vi "ncmainui.vi"() -> ()   [LabVIEW 2011]
uses:
  API/API DYM.lvlib
panel:
  in  "气缸":enum16{"向上", "向下"}(ring)
  in  "回参考点":bool
  out "CodeLine":i32
  out "CurrnetY":dbl
  out "CurrentX":dbl
  in  "撤消指令":bool
  in  "清空列表":bool
  in  "保存列表":bool
  in  "打开列表":bool
  in  "紧急停止":bool
  in  "开始执行":bool
  in  "选择坐标系统":enum32{"相对坐标", "绝度坐标"}(radio)
  in  "CodeList":i32(listbox)
  in  "G04DelayT":i32
  in  "G04":bool
  in  "G01z":dbl format="%.1f"
  in  "G01x":dbl format="%.1f"
  in  "G00z":dbl format="%.1f"
  in  "G00x":dbl format="%.1f"
  in  "G01":bool
  in  "G00":bool
  # "X(U):"
  # "Y(V):"
  # "mm"
  # "mm"
  # "X(U):"
  # "Y(V):"
  # "Z(W):"
  # "mm"
  # "mm"
  # "定时:"
  # "ms"
  # "当前位置坐标:"
  # "当前指令执行位置:"
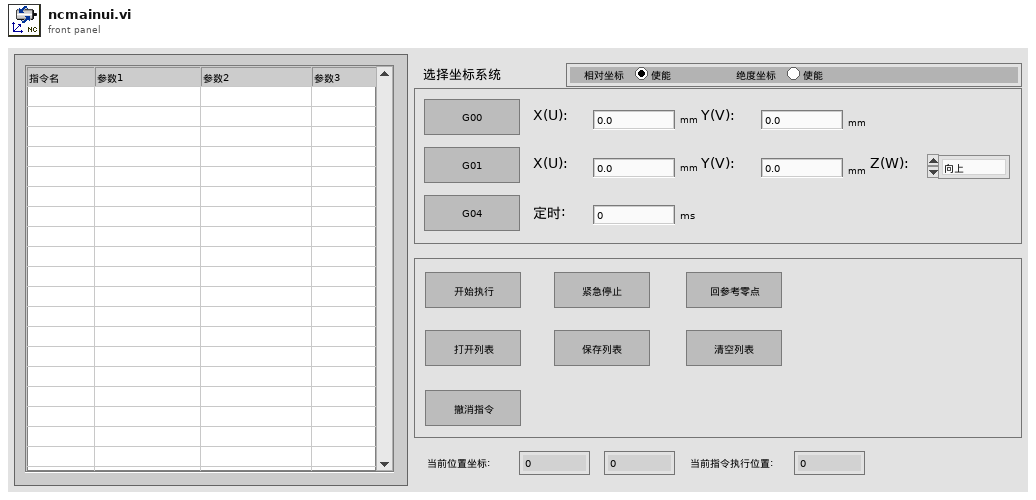
[diagram p1: front panel]
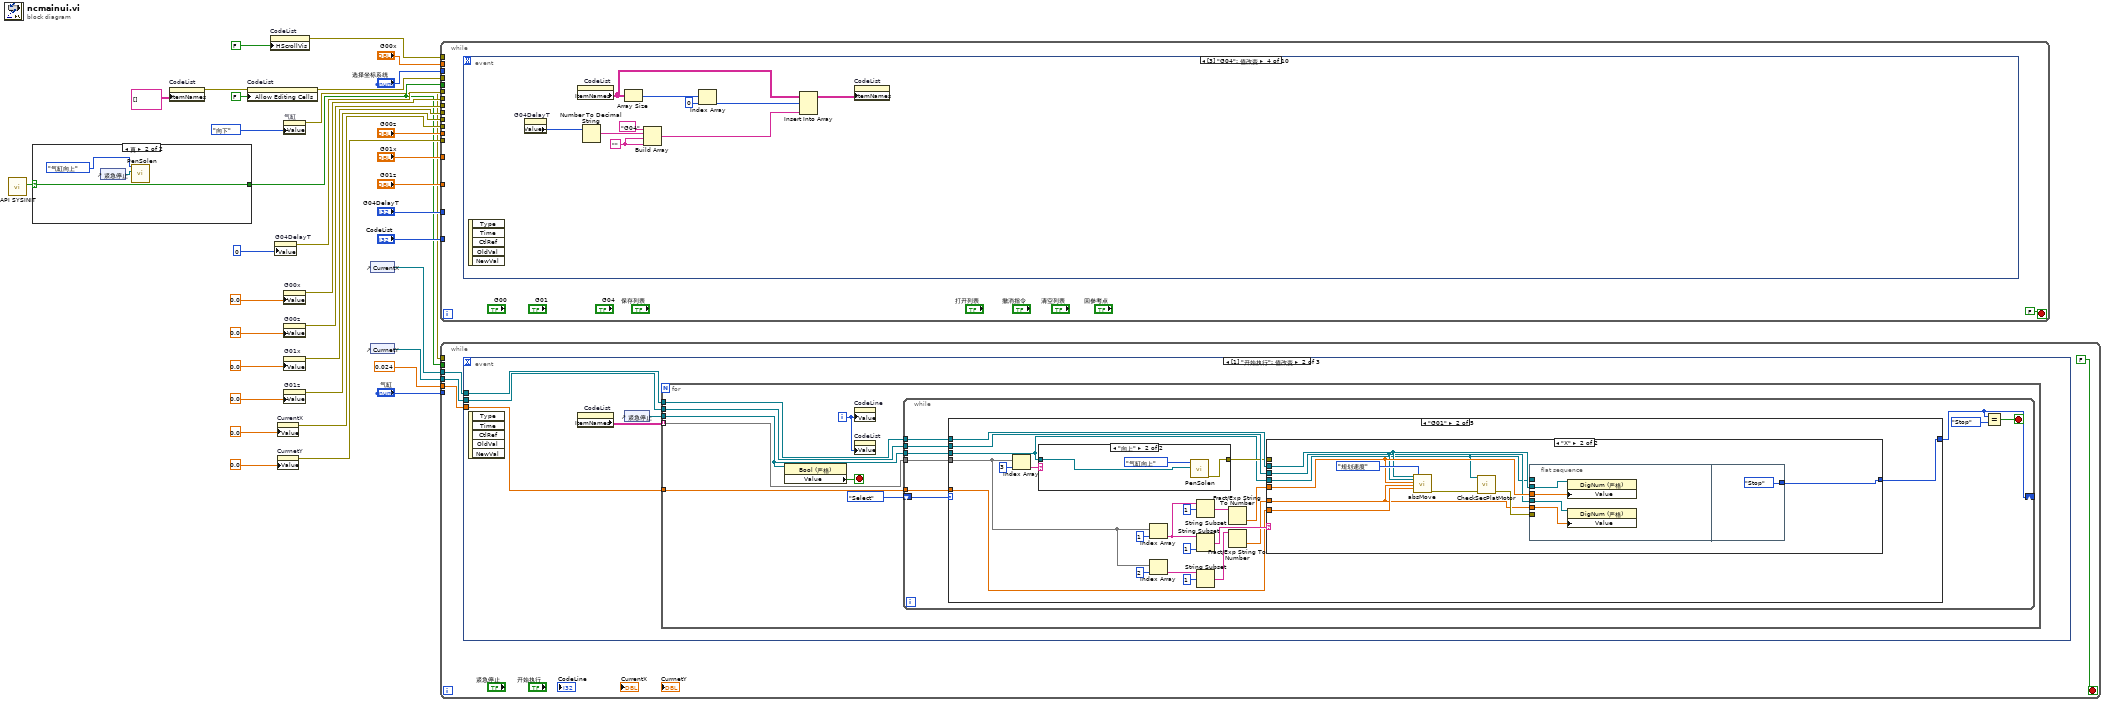
[diagram p0: block diagram]
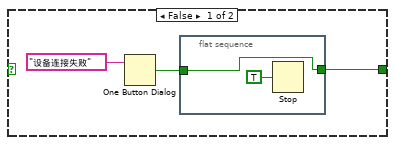
[diagram p2: hidden frame]
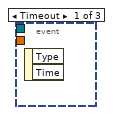
[diagram p3: hidden frame]
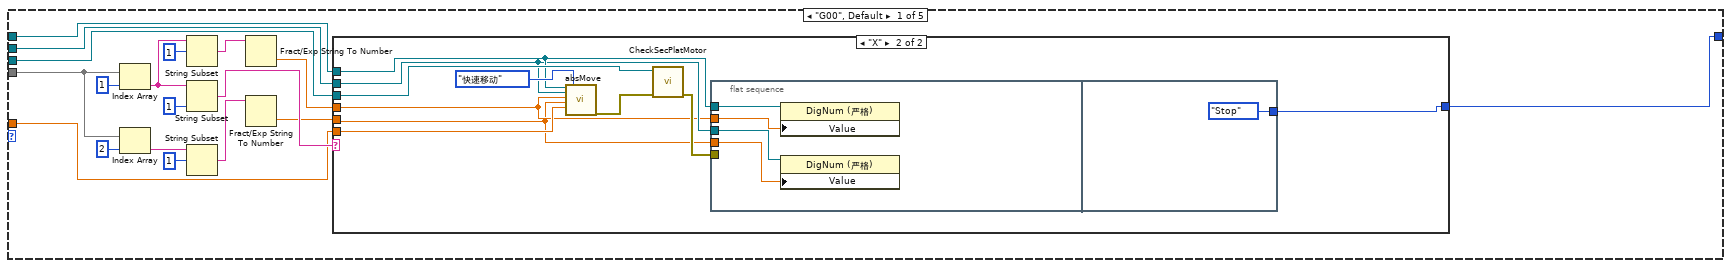
[diagram p4: hidden frame]
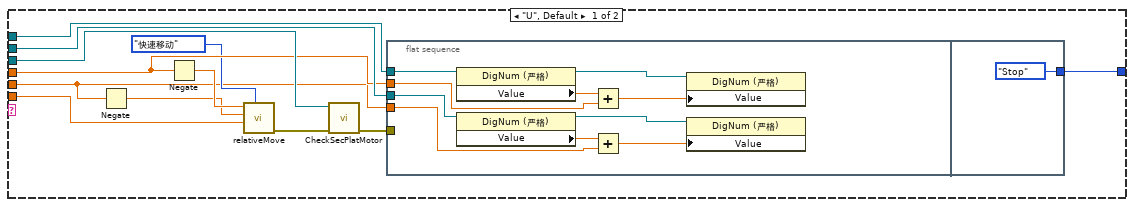
[diagram p5: hidden frame]
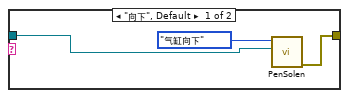
[diagram p6: hidden frame]
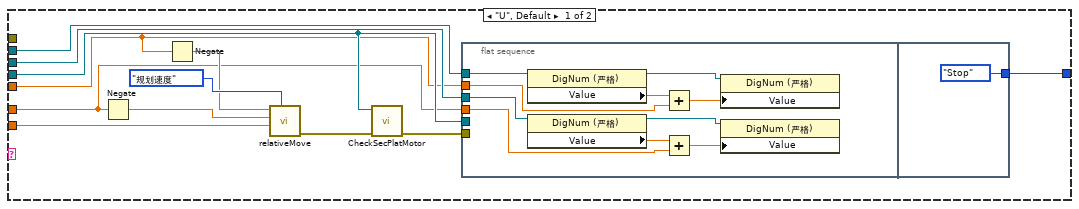
[diagram p7: hidden frame]
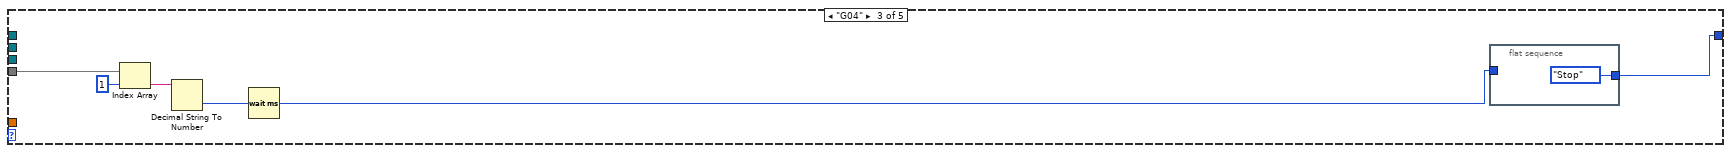
[diagram p8: hidden frame]
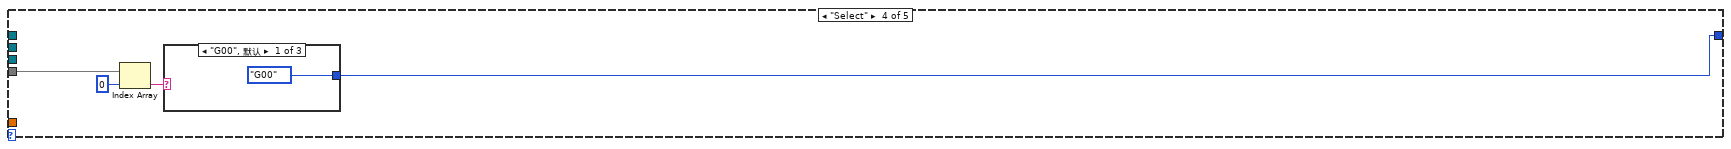
[diagram p9: hidden frame]
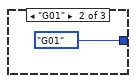
[diagram p10: hidden frame]
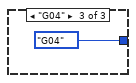
[diagram p11: hidden frame]
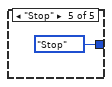
[diagram p12: hidden frame]
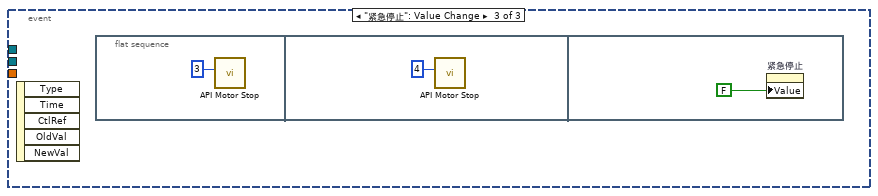
[diagram p13: hidden frame]
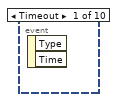
[diagram p14: hidden frame]
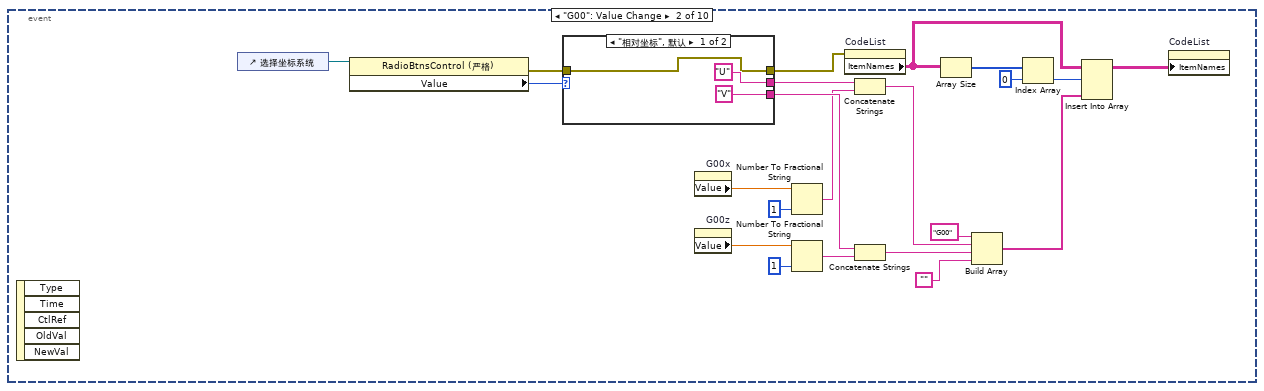
[diagram p15: hidden frame]
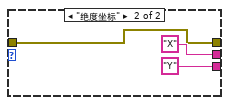
[diagram p16: hidden frame]
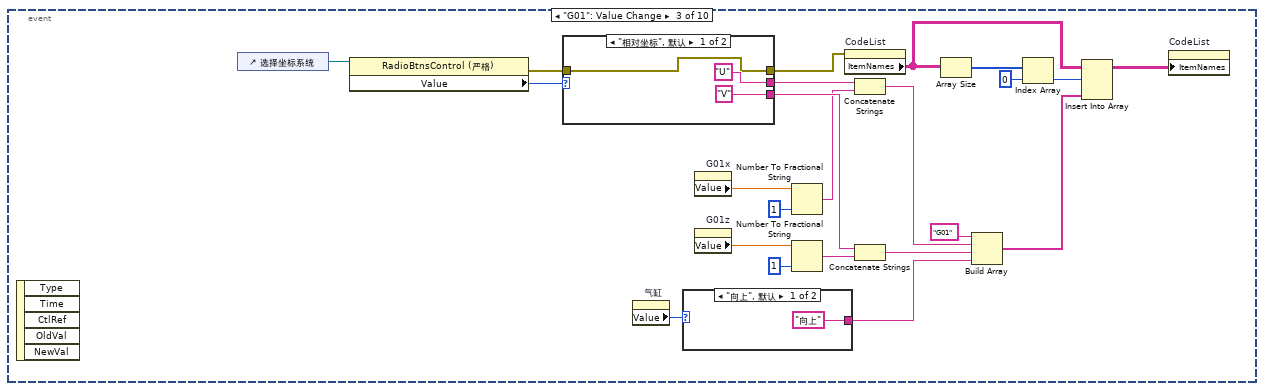
[diagram p17: hidden frame]
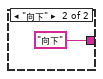
[diagram p18: hidden frame]
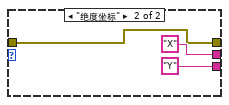
[diagram p19: hidden frame]
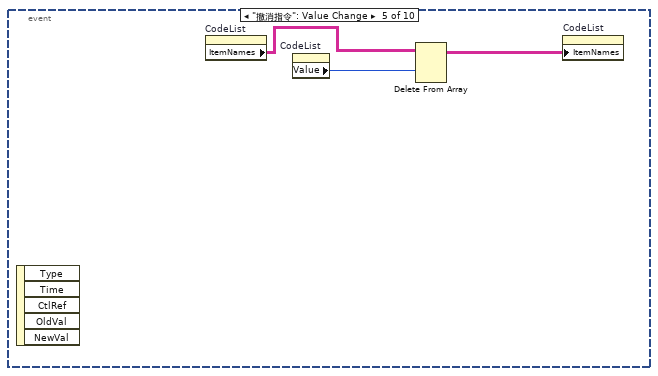
[diagram p20: hidden frame]
diagram:
  n1 = call "API SYSINIT.vi"() -> ("SYSINIT return value"=w5:bool)  [unwired: 11 in]
  n2 = case shown="真" w5 {
    selector: w5 -> [_ w41]
    tunnel: [w36 w41] -> w4
    frame False {
      n3 = One Button Dialog(message="设备连接失败" ("消息")) -> (true=w37:bool)  [unwired: 1 in]
      n4 = flat-sequence {
        tunnel: w37 -> [w39]
        tunnel: [w39] -> w36
        frame #0 {
          n5 = Stop(stop? (T)=TRUE ("停止？(T)")) -> ()
        }
      }
    }
    frame True {
      n6 = control-ref of="紧急停止"() -> (w42:refnum<vi>)
      n7 = call "PenSolen.vi"("Bool引用"=w42, "模式"=enum16{"气缸向下", "气缸向上"}."气缸向上") -> ()  [unwired: 9 in, 1 out]
    }
  }
  n8 = property on="CodeList" class="MCListbox (严格)"("ItemNames"=string[][] [] ("项名")) -> (error out=w10:errorcluster)  [unwired: 2 in, 1 out]
  n9 = property on="CodeList" class="MCListbox (严格)"(error in=w10, "Allow Editing Cells"=FALSE ("允许编辑单元格")) -> (error out=w13:errorcluster)  [unwired: 1 in, 1 out]
  n10 = property on="CodeList" class="MCListbox (严格)"("HScrollVis"=FALSE ("显示项:显示水平滚动条")) -> (error out=w11:errorcluster)  [unwired: 2 in, 1 out]
  n11 = property on="G04DelayT" class="DigNum (严格)"("Value"=0 ("G04DelayT")) -> (error out=w28:errorcluster)  [unwired: 2 in, 1 out]
  n12 = property on="CurrentX" class="DigNum (严格)"("Value"=0.0 ("CurrentX")) -> (error out=w16:errorcluster)  [unwired: 2 in, 1 out]
  n13 = property on="CurrnetY" class="DigNum (严格)"("Value"=0.0 ("CurrnetY")) -> (error out=w15:errorcluster)  [unwired: 2 in, 1 out]
  n14 = property on="气缸" class="Enum (严格)"("Value"=enum16{"向上", "向下"}."向下" ("气缸")) -> (error out=w1:errorcluster)  [unwired: 2 in, 1 out]
  n15 = property on="G00x" class="DigNum (严格)"("Value"=0.0 ("G00x")) -> (error out=w27:errorcluster)  [unwired: 2 in, 1 out]
  n16 = property on="G00z" class="DigNum (严格)"("Value"=0.0 ("G00z")) -> (error out=w26:errorcluster)  [unwired: 2 in, 1 out]
  n17 = property on="G01x" class="DigNum (严格)"("Value"=0.0 ("G01x")) -> (error out=w25:errorcluster)  [unwired: 2 in, 1 out]
  n18 = property on="G01z" class="DigNum (严格)"("Value"=0.0 ("G01z")) -> (error out=w24:errorcluster)  [unwired: 2 in, 1 out]
  n19 = control-ref of="CurrentX"() -> (w8:refnum<vi>)
  n20 = control-ref of="CurrnetY"() -> (w7:refnum<vi>)
  n21 = while {
    tunnel: "G00x" -> [_]
    tunnel: "G00z" -> [_]
    tunnel: "G01x" -> [_]
    tunnel: "G01z" -> [_]
    tunnel: "G04DelayT" -> [_]
    tunnel: "CodeList" -> [_]
    tunnel: "选择坐标系统" -> [_]
    tunnel: w28 -> [_]
    tunnel: w27 -> [_]
    tunnel: w26 -> [_]
    tunnel: w25 -> [_]
    tunnel: w24 -> [_]
    tunnel: w16 -> [_]
    tunnel: w15 -> [_]
    tunnel: w13 -> [_]
    tunnel: w11 -> [_]
    tunnel: w4 -> [_]
    stop <- FALSE stop-if-true
    n22 = event shown="[3] \"G04\": 值改变" {
      selector: _ -> [_ _ _ _ _ _ _ _ _ _]
      dyn-events: _ -> [_ _ _ _ _ _ _ _ _ _]
      timeout: _ -> [_ _ _ _ _ _ _ _ _ _]
      event Timeout {
        n23 = event-data() -> ()  [unwired: 1 in, 2 out]
      }
      event "G00": Value Change {
        n24 = event-data() -> ()  [unwired: 1 in, 5 out]
        n25 = control-ref of="选择坐标系统"() -> (w59:refnum<vi>)
        n26 = property class="RadioBtnsControl (严格)"(reference=w59) -> (error out=w47:errorcluster, "Value"=w58:enum32{"相对坐标", "绝度坐标"})  [unwired: 1 in, 1 out]
        n27 = case shown="\"相对坐标\", 默认" w58 {
          tunnel: ["U" "X"] -> w57
          tunnel: ["V" "Y"] -> w56
          tunnel: w47 -> [w67 w70]
          tunnel: [w67 w70] -> w46
          frame "相对坐标", Default {
          }
          frame "绝度坐标" {
          }
        }
        n28 = property on="G00x" class="DigNum (严格)"() -> ("Value"=w55:dbl)  [unwired: 2 in, 2 out]
        n29 = property on="G00z" class="DigNum (严格)"() -> ("Value"=w52:dbl)  [unwired: 2 in, 2 out]
        n30 = Number To Fractional String(number=w55, precision (6)=i16 1 ("精度(6)")) -> (F-format string=w53:string)  [unwired: 2 in]
        n31 = Number To Fractional String(number=w52, precision (6)=i16 1 ("精度(6)")) -> (F-format string=w50:string)  [unwired: 2 in]
        n32 = property on="CodeList" class="MCListbox (严格)"(error in=w46) -> ("ItemNames"=w64:string[][])  [unwired: 1 in, 2 out]
        n33 = Concatenate Strings(w57, w53) -> (w49:string)
        n34 = Concatenate Strings(w56, w50) -> (w48:string)
        n35 = Array Size(array=w64) -> (size(s)=w66:i32[])
        n36 = Build Array("G00", w49, w48, "") -> (w61:string[])
        n37 = Index Array(array=w66, index=0 ("索引")) -> (element=w63:i32)
        n38 = Insert Into Array(array=w64, index (row)=w63, new element=w61) -> (w60:string[][])  [unwired: 1 in]
        n39 = property on="CodeList" class="MCListbox (严格)"("ItemNames"=w60) -> ()  [unwired: 2 in, 2 out]
      }
      event "G01": Value Change {
        n40 = event-data() -> ()  [unwired: 1 in, 5 out]
        n41 = control-ref of="选择坐标系统"() -> (w88:refnum<vi>)
        n42 = property class="RadioBtnsControl (严格)"(reference=w88) -> (error out=w78:errorcluster, "Value"=w87:enum32{"相对坐标", "绝度坐标"})  [unwired: 1 in, 1 out]
        n43 = case shown="\"相对坐标\", 默认" w87 {
          tunnel: ["U" "X"] -> w86
          tunnel: ["V" "Y"] -> w85
          tunnel: w78 -> [w98 w101]
          tunnel: [w98 w101] -> w77
          frame "相对坐标", Default {
          }
          frame "绝度坐标" {
          }
        }
        n44 = property on="气缸" class="Enum (严格)"() -> ("Value"=w74:enum16{"向上", "向下"})  [unwired: 2 in, 2 out]
        n45 = case shown="\"向上\", 默认" w74 {
          tunnel: ["向上" "向下"] -> w73
          frame "向上", Default {
          }
          frame "向下" {
          }
        }
        n46 = property on="G01x" class="DigNum (严格)"() -> ("Value"=w76:dbl)  [unwired: 2 in, 2 out]
        n47 = property on="G01z" class="DigNum (严格)"() -> ("Value"=w75:dbl)  [unwired: 2 in, 2 out]
        n48 = Number To Fractional String(number=w76, precision (6)=i16 1 ("精度(6)")) -> (F-format string=w83:string)  [unwired: 2 in]
        n49 = Number To Fractional String(number=w75, precision (6)=i16 1 ("精度(6)")) -> (F-format string=w81:string)  [unwired: 2 in]
        n50 = property on="CodeList" class="MCListbox (严格)"(error in=w77) -> ("ItemNames"=w93:string[][])  [unwired: 1 in, 2 out]
        n51 = Concatenate Strings(w86, w83) -> (w80:string)
        n52 = Concatenate Strings(w85, w81) -> (w79:string)
        n53 = Array Size(array=w93) -> (size(s)=w95:i32[])
        n54 = Build Array("G01", w80, w79, w73) -> (w90:string[])
        n55 = Index Array(array=w95, index=0 ("索引")) -> (element=w92:i32)
        n56 = Insert Into Array(array=w93, index (row)=w92, new element=w90) -> (w89:string[][])  [unwired: 1 in]
        n57 = property on="CodeList" class="MCListbox (严格)"("ItemNames"=w89) -> ()  [unwired: 2 in, 2 out]
      }
      event "G04": Value Change {
        w104 = ""
        n58 = event-data() -> ()  [unwired: 1 in, 5 out]
        n59 = property on="G04DelayT" class="DigNum (严格)"() -> ("Value"=w106:i32)  [unwired: 2 in, 2 out]
        n60 = property on="CodeList" class="MCListbox (严格)"() -> ("ItemNames"=w111:string[][])  [unwired: 2 in, 2 out]
        n61 = Number To Decimal String(number=w106) -> (decimal integer string=w105:string)  [unwired: 1 in]
        n62 = Array Size(array=w111) -> (size(s)=w113:i32[])
        n63 = Build Array("G04", w105, w104, w104) -> (w108:string[])
        n64 = Index Array(array=w113, index=0 ("索引")) -> (element=w110:i32)
        n65 = Insert Into Array(array=w111, index (row)=w110, new element=w108) -> (w107:string[][])  [unwired: 1 in]
        n66 = property on="CodeList" class="MCListbox (严格)"("ItemNames"=w107) -> ()  [unwired: 2 in, 2 out]
      }
      event "撤消指令": Value Change {
        n67 = event-data() -> ()  [unwired: 1 in, 5 out]
        n68 = property on="CodeList" class="MCListbox (严格)"() -> ("ItemNames"=w116:string[][])  [unwired: 2 in, 2 out]
        n69 = property on="CodeList" class="MCListbox (严格)"() -> ("Value"=w115:i32)  [unwired: 2 in, 2 out]
        n70 = Delete From Array(array=w116, index (row)=w115) -> (array with subset deleted=w114:string[][])  [unwired: 2 in, 1 out]
        n71 = property on="CodeList" class="MCListbox (严格)"("ItemNames"=w114) -> ()  [unwired: 2 in, 2 out]
      }
      event "保存列表": Value Change {
        n72 = event-data() -> ()  [unwired: 1 in, 5 out]
        n73 = call "文件对话框_保存"("prompt"="保存文件", "button label"="保存", "pattern (all files)"="*.GCode", "pattern label"="G代码") -> ("selected path"=w117:path, "error out"=w118:errorcluster)  [unwired: 8 in, 2 out]
        n74 = case shown="无错误" w118 {
          selector: w118 -> [_ w136]
          tunnel: w117 -> [w124 _]
          frame No Error {
            n75 = property on="CodeList" class="MCListbox (严格)"() -> ("ItemNames"=w126:string[][])  [unwired: 2 in, 2 out]
            n76 = for {
              tunnel: w126 -> [w131] mode=indexing
              shift-right: [w128] -> w123
              shift-left: "" -> [w130]
              n77 = for {
                tunnel: w131 -> [w134] mode=indexing
                shift-right: [w133] -> w127
                shift-left: w130 -> [w135]
                n78 = call <vilib>:"Space Constant.vi"() -> ("String"=w132:string)
                n79 = Concatenate Strings(w135, w134, w132) -> (w133:string)
              }
              n80 = Concatenate Strings(w127, "\n") -> (w128:string)
            }
            n81 = Write to Text File(file (use dialog)=w124, text=w123) -> ()  [unwired: 2 in, 3 out]
          }
          frame Error {
            n82 = call <vilib>:"Clear Errors.vi"("error in (no error)"=w136) -> ()  [unwired: 6 in, 1 out]
          }
        }
      }
      event "清空列表": Value Change {
        n83 = event-data() -> ()  [unwired: 1 in, 5 out]
        n84 = property on="CodeList" class="MCListbox (严格)"("ItemNames"=string[][] [] ("项名")) -> ()  [unwired: 2 in, 2 out]
      }
      event "打开列表": Value Change {
        n85 = event-data() -> ()  [unwired: 1 in, 5 out]
        n86 = call "文件对话框_打开"("prompt"="打开文件", "button label"="打开", "pattern (all files)"="*.GCode", "pattern label"="G代码") -> ("selected path"=w138:path, "error out"=w139:errorcluster)  [unwired: 8 in, 2 out]
        n87 = case shown="无错误" w139 {
          selector: w139 -> [_ w190]
          tunnel: w138 -> [w149 _]
          frame No Error {
            n88 = Read from Text File(file (use dialog)=w149, count=-1 ("计数")) -> (text=w147:string[])  [unwired: 2 in, 3 out]
            n89 = Initialize Array("") -> (w145:string[][])  [unwired: 2 in]
            n90 = for {
              tunnel: w147 -> [w155] mode=indexing
              shift-right: [w151] -> w144
              shift-left: w145 -> [w153]
              i -> [w152]
              n91 = String Subset(string=w155, length (rest)=3 ("长度（剩余）")) -> (substring=w154:string)  [unwired: 1 in]
              n92 = case shown="\"G01\"" w154 {
                tunnel: w155 -> [w162 w168 w181]
                tunnel: w154 -> [w163 w165 w182]
                tunnel: [w157 w164 w180] -> w150
                frame "G04" {
                  n93 = String Subset(string=w162, offset (0)=4 ("偏移量(0)")) -> (substring=w160:string)  [unwired: 1 in]
                  n94 = call <vilib>:"Space Constant.vi"() -> ("String"=w159:string)
                  n95 = Search/Split String(string=w160, search string/char (-)=w159) -> (substring before match=w158:string)  [unwired: 1 in, 2 out]
                  n96 = Build Array(w163, w158) -> (w157:string[])
                }
                frame "G00", Default {
                  n97 = String Subset(string=w168, offset (0)=4 ("偏移量(0)")) -> (substring=w170:string)  [unwired: 1 in]
                  n98 = call <vilib>:"Space Constant.vi"() -> ("String"=w174:string)
                  n99 = Search/Split String(string=w170, search string/char (-)=w174) -> (substring before match=w166:string, match + rest of string=w171:string)  [unwired: 1 in, 1 out]
                  n100 = String Subset(string=w171, offset (0)=1 ("偏移量(0)")) -> (substring=w173:string)  [unwired: 1 in]
                  n101 = Search/Split String(string=w173, search string/char (-)=w174) -> (substring before match=w167:string)  [unwired: 1 in, 2 out]
                  n102 = Build Array(w165, w166, w167) -> (w164:string[])
                }
                frame "G01" {
                  n103 = String Subset(string=w181, offset (0)=4 ("偏移量(0)")) -> (substring=w186:string)  [unwired: 1 in]
                  n104 = call <vilib>:"Space Constant.vi"() -> ("String"=w176:string)
                  n105 = Search/Split String(string=w186, search string/char (-)=w176) -> (substring before match=w183:string, match + rest of string=w187:string)  [unwired: 1 in, 1 out]
                  n106 = String Subset(string=w187, offset (0)=1 ("偏移量(0)")) -> (substring=w189:string)  [unwired: 1 in]
                  n107 = Search/Split String(string=w189, search string/char (-)=w176) -> (substring before match=w184:string, match + rest of string=w179:string)  [unwired: 1 in, 1 out]
                  n108 = String Subset(string=w179, offset (0)=1 ("偏移量(0)")) -> (substring=w177:string)  [unwired: 1 in]
                  n109 = Search/Split String(string=w177, search string/char (-)=w176) -> (substring before match=w175:string)  [unwired: 1 in, 2 out]
                  n110 = Build Array(w182, w183, w184, w175) -> (w180:string[])
                }
              }
              n111 = Insert Into Array(array=w153, index (row)=w152, new element=w150) -> (w151:string[][])  [unwired: 1 in]
            }
            n112 = property on="CodeList" class="MCListbox (严格)"("ItemNames"=w144) -> ()  [unwired: 2 in, 2 out]
          }
          frame Error {
            n113 = call <vilib>:"Clear Errors.vi"("error in (no error)"=w190) -> ()  [unwired: 6 in, 1 out]
          }
        }
      }
      event "回参考点": Value Change {
        n114 = event-data() -> ()  [unwired: 1 in, 5 out]
        n115 = flat-sequence {
          frame #0 {
            n116 = control-ref of="紧急停止"() -> (w191:refnum<vi>)
            n117 = call "PenSolen.vi"("Bool引用"=w191, "模式"=enum16{"气缸向下", "气缸向上"}."气缸向上") -> ()  [unwired: 9 in, 1 out]
          }
          frame #1 {
            n118 = call "API Set Motor Speed.vi"("motorSpeed"=1500, "motorNum"=3) -> ()  [unwired: 9 in, 1 out]
          }
          frame #2 {
            n119 = call "API Set Motor Speed.vi"("motorSpeed"=1500, "motorNum"=4) -> ()  [unwired: 9 in, 1 out]
          }
          frame #3 {
            n120 = call "API Motor Start.vi"("stepNum"=40000, "direction"=1, "motorNum"=3) -> ()  [unwired: 8 in, 1 out]
          }
          frame #4 {
            n121 = call "API Motor Start.vi"("stepNum"=40000, "direction"=1, "motorNum"=4) -> ()  [unwired: 8 in, 1 out]
          }
          frame #5 {
            n122 = control-ref of="紧急停止"() -> (w203:refnum<vi>)
            n123 = call "CheckSecPlatMotor.vi"("Bool引用"=w203) -> ()  [unwired: 10 in, 1 out]
          }
          frame #6 {
            n124 = call "API Motor Start.vi"("stepNum"=8100, "direction"=0, "motorNum"=3) -> ()  [unwired: 8 in, 1 out]
          }
          frame #7 {
            n125 = call "API Motor Start.vi"("stepNum"=3700, "direction"=0, "motorNum"=4) -> ()  [unwired: 8 in, 1 out]
          }
          frame #8 {
            n126 = control-ref of="紧急停止"() -> (w210:refnum<vi>)
            n127 = call "CheckSecPlatMotor.vi"("Bool引用"=w210) -> ()  [unwired: 10 in, 1 out]
          }
          frame #9 {
            n128 = property on="CurrentX" class="DigNum (严格)"("Value"=0.0 ("CurrentX")) -> ()  [unwired: 2 in, 2 out]
            n129 = property on="CurrnetY" class="DigNum (严格)"("Value"=0.0 ("CurrnetY")) -> ()  [unwired: 2 in, 2 out]
          }
        }
      }
      event Panel Close {
        n130 = event-data() -> ()  [unwired: 1 in, 3 out]
        n131 = call "API SYSQUIT.vi"() -> ()  [unwired: 12 in]
      }
    }
  }
  n132 = while {
    tunnel: w8 -> [w215]
    tunnel: w7 -> [w214]
    tunnel: 0.024 -> [w213]
    tunnel: w4 -> [_]
    tunnel: "气缸" -> [_]
    tunnel: w1 -> [_]
    stop <- FALSE stop-if-true
    n133 = event shown="[1] \"开始执行\": 值改变" {
      selector: _ -> [_ _ _]
      dyn-events: _ -> [_ _ _]
      timeout: _ -> [_ _ _]
      tunnel: w215 -> [_ w220 _]
      tunnel: w214 -> [_ w219 _]
      tunnel: w213 -> [_ w218 _]
      event Timeout {
        n134 = event-data() -> ()  [unwired: 1 in, 2 out]
      }
      event "开始执行": Value Change {
        n135 = event-data() -> ()  [unwired: 1 in, 5 out]
        n136 = property on="CodeList" class="MCListbox (严格)"() -> ("ItemNames"=w221:string[][])  [unwired: 2 in, 2 out]
        n137 = control-ref of="紧急停止"() -> (w217:refnum<vi>)
        n138 = for {
          tunnel: w221 -> [w228] mode=indexing
          tunnel: w220 -> [w227]
          tunnel: w219 -> [w226]
          tunnel: w218 -> [w225]
          tunnel: w217 -> [w224]
          i -> [w222]
          stop <- w223 stop-if-true
          n139 = property class="Bool (严格)"(reference=w224) -> ("Value"=w223:bool)  [unwired: 1 in, 2 out]
          n140 = property on="CodeLine" class="DigNum (严格)"("Value"=w222) -> ()  [unwired: 2 in, 2 out]
          n141 = property on="CodeList" class="MCListbox (严格)"("Value"=w222) -> ()  [unwired: 2 in, 2 out]
          n142 = while {
            shift-right: [w232] -> _
            shift-left: enum16{"G00", "G01", "G04", "Select", "Stop"}."Select" -> [w238]
            tunnel: w228 -> [w237]
            tunnel: w227 -> [w236]
            tunnel: w226 -> [w235]
            tunnel: w225 -> [w234]
            tunnel: w224 -> [w233]
            stop <- w230 stop-if-true
            n143 = case shown="\"G01\"" w238 {
              tunnel: w237 -> [w255 w299 w365 w370 _]
              tunnel: [w239 w300 w360 w367 enum16{"G00", "G01", "G04", "Select", "Stop"}."Stop"] -> w232
              tunnel: w236 -> [w243 w302 _ _ _]
              tunnel: w235 -> [w242 w301 _ _ _]
              tunnel: w234 -> [w241 w303 _ _ _]
              tunnel: w233 -> [w240 w295 _ _ _]
              frame "G00", Default {
                n144 = Index Array(array=w255, index=1 ("索引")) -> (element=w251:string)
                n145 = Index Array(array=w255, index=2 ("索引")) -> (element=w249:string)
                n146 = String Subset(string=w251, offset (0)=1 ("偏移量(0)")) -> (substring=w247:string)  [unwired: 1 in]
                n147 = String Subset(string=w251, length (rest)=1 ("长度（剩余）")) -> (substring=w252:string)  [unwired: 1 in]
                n148 = String Subset(string=w249, offset (0)=1 ("偏移量(0)")) -> (substring=w245:string)  [unwired: 1 in]
                n149 = Fract/Exp String To Number(string=w247) -> (number=w246:dbl)  [unwired: 3 in, 1 out]
                n150 = Fract/Exp String To Number(string=w245) -> (number=w244:dbl)  [unwired: 3 in, 1 out]
                n151 = case shown="\"X\"" w252 {
                  tunnel: w246 -> [w261 w282]
                  tunnel: w244 -> [w258 w281]
                  tunnel: w243 -> [w263 w284]
                  tunnel: w242 -> [w262 w283]
                  tunnel: w241 -> [w268 w289]
                  tunnel: w240 -> [w266 w286]
                  tunnel: [w264 w280] -> w239
                  frame "U", Default {
                    n152 = Negate(x=w258) -> (-x=w257:dbl)
                    n153 = Negate(x=w261) -> (-x=w260:dbl)
                    n154 = call "relativeMove.vi"("模式"=enum16{"快速移动", "规划速度"}."快速移动", "Param_StepDis"=w268, "TargetY"=w257, "TargetX"=w260) -> ("错误输出"=w267:errorcluster)  [unwired: 7 in]
                    n155 = call "CheckSecPlatMotor.vi"("错误输入（无错误）"=w267, "Bool引用"=w266) -> ("错误输出"=w265:errorcluster)  [unwired: 9 in]
                    n156 = flat-sequence {
                      tunnel: w265 -> [_]
                      tunnel: w263 -> [w278]
                      tunnel: w262 -> [w277]
                      tunnel: w261 -> [w275]
                      tunnel: w258 -> [w274]
                      tunnel: [enum16{"G00", "G01", "G04", "Select", "Stop"}."Stop"] -> w264
                      frame #0 {
                        n157 = property class="DigNum (严格)"(reference=w278) -> (reference out=w270:refnum<vi>, "Value"=w276:dbl)  [unwired: 1 in, 1 out]
                        n158 = property class="DigNum (严格)"(reference=w277) -> (reference out=w269:refnum<vi>, "Value"=w273:dbl)  [unwired: 1 in, 1 out]
                        n159 = Add(x=w276, y=w275) -> (x+y=w271:dbl)
                        n160 = Add(x=w273, y=w274) -> (x+y=w272:dbl)
                        n161 = property class="DigNum (严格)"(reference=w270, "Value"=w271) -> ()  [unwired: 1 in, 2 out]
                        n162 = property class="DigNum (严格)"(reference=w269, "Value"=w272) -> ()  [unwired: 1 in, 2 out]
                      }
                      frame #1 {
                      }
                    }
                  }
                  frame "X" {
                    n163 = call "absMove.vi"("CurrentX引用"=w284, "CurrentY引用"=w283, "TargetX"=w282, "TargetY"=w281, "Param_StepDis"=w289, "模式"=enum16{"快速移动", "规划速度"}."快速移动") -> ("错误输出"=w287:errorcluster)  [unwired: 13 in]
                    n164 = call "CheckSecPlatMotor.vi"("错误输入（无错误）"=w287, "Bool引用"=w286) -> ("错误输出"=w285:errorcluster)  [unwired: 9 in]
                    n165 = flat-sequence {
                      tunnel: w285 -> [_]
                      tunnel: w284 -> [w293]
                      tunnel: w283 -> [w292]
                      tunnel: w282 -> [w291]
                      tunnel: w281 -> [w290]
                      tunnel: [enum16{"G00", "G01", "G04", "Select", "Stop"}."Stop"] -> w280
                      frame #0 {
                        n166 = property class="DigNum (严格)"(reference=w293, "Value"=w291) -> ()  [unwired: 1 in, 2 out]
                        n167 = property class="DigNum (严格)"(reference=w292, "Value"=w290) -> ()  [unwired: 1 in, 2 out]
                      }
                      frame #1 {
                      }
                    }
                  }
                }
              }
              frame "G01" {
                n168 = Index Array(array=w299, index=3 ("索引")) -> (element=w297:string)
                n169 = case shown="\"向上\"" w297 {
                  tunnel: [w318 w321] -> w296
                  tunnel: w295 -> [w316 w320]
                  frame "向下", Default {
                    n170 = call "PenSolen.vi"("Bool引用"=w316, "模式"=enum16{"气缸向下", "气缸向上"}."气缸向下") -> ("error out"=w318:errorcluster)  [unwired: 9 in]
                  }
                  frame "向上" {
                    n171 = call "PenSolen.vi"("Bool引用"=w320, "模式"=enum16{"气缸向下", "气缸向上"}."气缸向上") -> ("error out"=w321:errorcluster)  [unwired: 9 in]
                  }
                }
                n172 = Index Array(array=w299, index=1 ("索引")) -> (element=w312:string)
                n173 = Index Array(array=w299, index=2 ("索引")) -> (element=w310:string)
                n174 = String Subset(string=w312, offset (0)=1 ("偏移量(0)")) -> (substring=w308:string)  [unwired: 1 in]
                n175 = String Subset(string=w312, length (rest)=1 ("长度（剩余）")) -> (substring=w306:string)  [unwired: 1 in]
                n176 = String Subset(string=w310, offset (0)=1 ("偏移量(0)")) -> (substring=w307:string)  [unwired: 1 in]
                n177 = Fract/Exp String To Number(string=w308) -> (number=w305:dbl)  [unwired: 3 in, 1 out]
                n178 = Fract/Exp String To Number(string=w307) -> (number=w304:dbl)  [unwired: 3 in, 1 out]
                n179 = case shown="\"X\"" w306 {
                  tunnel: w305 -> [w325 w350]
                  tunnel: w304 -> [w323 w349]
                  tunnel: w302 -> [w329 w348]
                  tunnel: w301 -> [w328 w347]
                  tunnel: w303 -> [w333 w354]
                  tunnel: w295 -> [w326 w346]
                  tunnel: [w330 w345] -> w300
                  tunnel: w296 -> [_ _]
                  frame "U", Default {
                    n180 = Negate(x=w323) -> (-x=w322:dbl)
                    n181 = Negate(x=w325) -> (-x=w324:dbl)
                    n182 = call "relativeMove.vi"("模式"=enum16{"快速移动", "规划速度"}."规划速度", "Param_StepDis"=w333, "TargetY"=w322, "TargetX"=w324) -> ("错误输出"=w332:errorcluster)  [unwired: 7 in]
                    n183 = call "CheckSecPlatMotor.vi"("错误输入（无错误）"=w332, "Bool引用"=w326) -> ("错误输出"=w331:errorcluster)  [unwired: 9 in]
                    n184 = flat-sequence {
                      tunnel: w331 -> [_]
                      tunnel: w329 -> [w343]
                      tunnel: w328 -> [w342]
                      tunnel: w325 -> [w340]
                      tunnel: w323 -> [w339]
                      tunnel: w326 -> [_]
                      tunnel: [enum16{"G00", "G01", "G04", "Select", "Stop"}."Stop"] -> w330
                      frame #0 {
                        n185 = property class="DigNum (严格)"(reference=w343) -> (reference out=w335:refnum<vi>, "Value"=w341:dbl)  [unwired: 1 in, 1 out]
                        n186 = property class="DigNum (严格)"(reference=w342) -> (reference out=w334:refnum<vi>, "Value"=w338:dbl)  [unwired: 1 in, 1 out]
                        n187 = Add(x=w341, y=w340) -> (x+y=w336:dbl)
                        n188 = Add(x=w338, y=w339) -> (x+y=w337:dbl)
                        n189 = property class="DigNum (严格)"(reference=w335, "Value"=w336) -> ()  [unwired: 1 in, 2 out]
                        n190 = property class="DigNum (严格)"(reference=w334, "Value"=w337) -> ()  [unwired: 1 in, 2 out]
                      }
                      frame #1 {
                      }
                    }
                  }
                  frame "X" {
                    n191 = call "absMove.vi"("CurrentX引用"=w348, "CurrentY引用"=w347, "TargetX"=w350, "TargetY"=w349, "Param_StepDis"=w354, "模式"=enum16{"快速移动", "规划速度"}."规划速度") -> ("错误输出"=w353:errorcluster)  [unwired: 13 in]
                    n192 = call "CheckSecPlatMotor.vi"("错误输入（无错误）"=w353, "Bool引用"=w346) -> ("错误输出"=w351:errorcluster)  [unwired: 9 in]
                    n193 = flat-sequence {
                      tunnel: w346 -> [_]
                      tunnel: w347 -> [w355]
                      tunnel: w348 -> [w356]
                      tunnel: w349 -> [w357]
                      tunnel: w350 -> [w358]
                      tunnel: w351 -> [_]
                      tunnel: [enum16{"G00", "G01", "G04", "Select", "Stop"}."Stop"] -> w345
                      frame #0 {
                        n194 = property class="DigNum (严格)"(reference=w356, "Value"=w358) -> ()  [unwired: 1 in, 2 out]
                        n195 = property class="DigNum (严格)"(reference=w355, "Value"=w357) -> ()  [unwired: 1 in, 2 out]
                      }
                      frame #1 {
                      }
                    }
                  }
                }
              }
              frame "G04" {
                n196 = Index Array(array=w365, index=1 ("索引")) -> (element=w363:string)
                n197 = Decimal String To Number(string=w363) -> (number=w362:i32)  [unwired: 2 in, 1 out]
                n198 = Wait (ms)(milliseconds to wait=w362) -> (millisecond timer value=w361:u32)
                n199 = flat-sequence {
                  tunnel: w361 -> [_]
                  tunnel: [enum16{"G00", "G01", "G04", "Select", "Stop"}."Stop"] -> w360
                  frame #0 {
                  }
                }
              }
              frame "Select" {
                n200 = Index Array(array=w370, index=0 ("索引")) -> (element=w368:string)
                n201 = case shown="\"G00\", 默认" w368 {
                  tunnel: [enum16{"G00", "G01", "G04", "Select", "Stop"}."G00" enum16{"G00", "G01", "G04", "Select", "Stop"}."G01" enum16{"G00", "G01", "G04", "Select", "Stop"}."G04"] -> w367
                  frame "G00", Default {
                  }
                  frame "G01" {
                  }
                  frame "G04" {
                  }
                }
              }
              frame "Stop" {
              }
            }
            n202 = Equal?(x=w232, y=enum16{"G00", "G01", "G04", "Select", "Stop"}."Stop") -> (x = y?=w230:bool)
          }
        }
      }
      event "紧急停止": Value Change {
        n203 = event-data() -> ()  [unwired: 1 in, 5 out]
        n204 = flat-sequence {
          frame #0 {
            n205 = call "API Motor Stop.vi"("motorNum"=3) -> ()  [unwired: 10 in, 1 out]
          }
          frame #1 {
            n206 = call "API Motor Stop.vi"("motorNum"=4) -> ()  [unwired: 10 in, 1 out]
          }
          frame #2 {
            n207 = property on="紧急停止" class="Bool (严格)"("Value"=FALSE ("紧急停止")) -> ()  [unwired: 2 in, 2 out]
          }
        }
      }
    }
  }
